vi "Set Current Range in Sweep - Binary Search.vi"(0 "VISA resource name":refnum<visa-resource-name>="GPIB0::24::INSTR", 5 "R":i32, 11 "error in (no error)":errorcluster) -> (4 "VISA resource name out":refnum<visa-resource-name>="GPIB0::24::INSTR", 15 "error out":errorcluster)   [LabVIEW 2010]
uses:
  <instrlib>/Keithley 2400/Keithley 24XX.lvlib
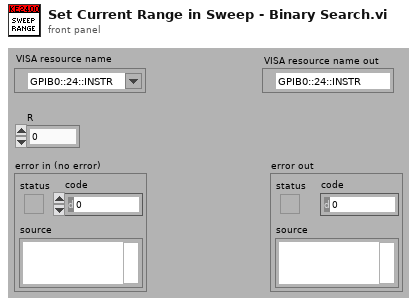
[diagram p1: front panel]
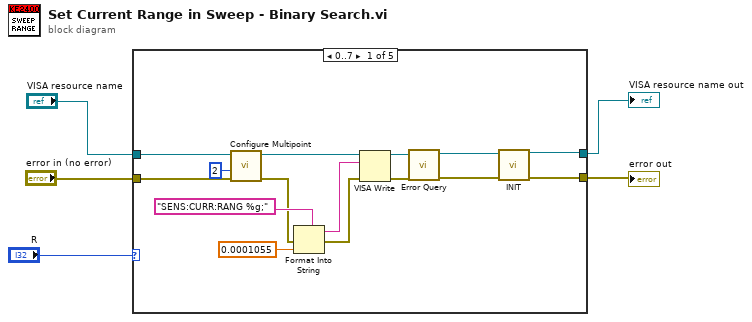
[diagram p0: block diagram]
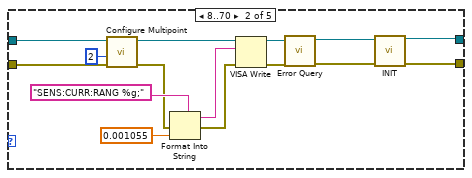
[diagram p2: hidden frame]
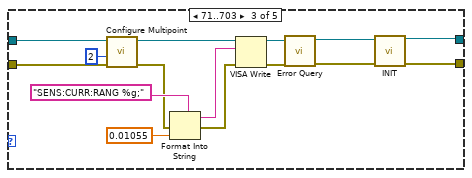
[diagram p3: hidden frame]
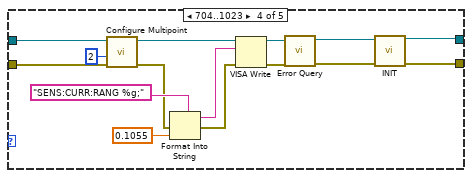
[diagram p4: hidden frame]
diagram:
  n1 = case shown="0..7" "R" {
    tunnel: [w15 w30 w45 w60 w67] -> w5
    tunnel: [w17 w32 w47 w62 w66] -> w4
    tunnel: "VISA resource name" -> [w10 w22 w37 w52 w67]
    tunnel: "error in (no error)" -> [w9 w21 w36 w51 w66]
    frame 0..7 {
      n2 = call <instrlib>:"Configure Multipoint.vi"("error in (no error)"=w9, "Trigger Count (1)"=2, "VISA resource name"=w10) -> ("error out"=w8:errorcluster, "VISA resource name out"=w7:refnum<visa-resource-name>)  [unwired: 7 in]
      n3 = Format Into String(format string="SENS:CURR:RANG %g;" ("Manual Range"), error in=w8, 0.0001055 ("R 2")) -> (resulting string=w12:string, error out=w11:errorcluster)  [unwired: 1 in]
      n4 = VISA Write(VISA resource name=w7, write buffer=w12, error in (no error)=w11) -> (VISA resource name out=w19:refnum<visa-resource-name>, error out=w18:errorcluster)  [unwired: 1 out]
      n5 = call <instrlib>:"Error Query.vi"("error in (no error)"=w18, "VISA resource name"=w19) -> ("error out"=w20:errorcluster, "VISA resource name out"=w16:refnum<visa-resource-name>)  [unwired: 6 in, 2 out]
      n6 = call "INIT.vi"("VISA resource name"=w16, "error in (no error)"=w20) -> ("VISA resource name out"=w15:refnum<visa-resource-name>, "error out"=w17:errorcluster)  [unwired: 12 in]
    }
    frame 8..70 {
      n7 = call <instrlib>:"Configure Multipoint.vi"("error in (no error)"=w21, "Trigger Count (1)"=2, "VISA resource name"=w22) -> ("error out"=w25:errorcluster, "VISA resource name out"=w24:refnum<visa-resource-name>)  [unwired: 7 in]
      n8 = Format Into String(format string="SENS:CURR:RANG %g;" ("Manual Range"), error in=w25, 0.001055 ("R 2")) -> (resulting string=w27:string, error out=w26:errorcluster)  [unwired: 1 in]
      n9 = VISA Write(VISA resource name=w24, write buffer=w27, error in (no error)=w26) -> (VISA resource name out=w34:refnum<visa-resource-name>, error out=w33:errorcluster)  [unwired: 1 out]
      n10 = call <instrlib>:"Error Query.vi"("error in (no error)"=w33, "VISA resource name"=w34) -> ("error out"=w35:errorcluster, "VISA resource name out"=w31:refnum<visa-resource-name>)  [unwired: 6 in, 2 out]
      n11 = call "INIT.vi"("VISA resource name"=w31, "error in (no error)"=w35) -> ("VISA resource name out"=w30:refnum<visa-resource-name>, "error out"=w32:errorcluster)  [unwired: 12 in]
    }
    frame 71..703 {
      n12 = call <instrlib>:"Configure Multipoint.vi"("error in (no error)"=w36, "Trigger Count (1)"=2, "VISA resource name"=w37) -> ("error out"=w40:errorcluster, "VISA resource name out"=w39:refnum<visa-resource-name>)  [unwired: 7 in]
      n13 = Format Into String(format string="SENS:CURR:RANG %g;" ("Manual Range"), error in=w40, 0.01055 ("R 2")) -> (resulting string=w42:string, error out=w41:errorcluster)  [unwired: 1 in]
      n14 = VISA Write(VISA resource name=w39, write buffer=w42, error in (no error)=w41) -> (VISA resource name out=w49:refnum<visa-resource-name>, error out=w48:errorcluster)  [unwired: 1 out]
      n15 = call <instrlib>:"Error Query.vi"("error in (no error)"=w48, "VISA resource name"=w49) -> ("error out"=w50:errorcluster, "VISA resource name out"=w46:refnum<visa-resource-name>)  [unwired: 6 in, 2 out]
      n16 = call "INIT.vi"("VISA resource name"=w46, "error in (no error)"=w50) -> ("VISA resource name out"=w45:refnum<visa-resource-name>, "error out"=w47:errorcluster)  [unwired: 12 in]
    }
    frame 704..1023 {
      n17 = call <instrlib>:"Configure Multipoint.vi"("error in (no error)"=w51, "Trigger Count (1)"=2, "VISA resource name"=w52) -> ("error out"=w55:errorcluster, "VISA resource name out"=w54:refnum<visa-resource-name>)  [unwired: 7 in]
      n18 = Format Into String(format string="SENS:CURR:RANG %g;" ("Manual Range"), error in=w55, 0.1055 ("R 2")) -> (resulting string=w57:string, error out=w56:errorcluster)  [unwired: 1 in]
      n19 = VISA Write(VISA resource name=w54, write buffer=w57, error in (no error)=w56) -> (VISA resource name out=w64:refnum<visa-resource-name>, error out=w63:errorcluster)  [unwired: 1 out]
      n20 = call <instrlib>:"Error Query.vi"("error in (no error)"=w63, "VISA resource name"=w64) -> ("error out"=w65:errorcluster, "VISA resource name out"=w61:refnum<visa-resource-name>)  [unwired: 6 in, 2 out]
      n21 = call "INIT.vi"("VISA resource name"=w61, "error in (no error)"=w65) -> ("VISA resource name out"=w60:refnum<visa-resource-name>, "error out"=w62:errorcluster)  [unwired: 12 in]
    }
    frame 1024, Default {
    }
  }
  "VISA resource name out" <- w5
  "error out" <- w4
